vi "Startup Panel.vi"() -> (0 "Bool Out":bool, 1 "ROV Selector Out":u16, 2 "Port Number Recv Out 1":u16, 3 "IP Address Out":string, 4 "Restart Out":bool, 6 "Port Number  Send Out":u16, 8 "Port Number Joyst. Out":u16)   [LabVIEW 2014]
uses:
  <vilib>/Platform/TimedLoop/XDataNode/timing_clust.ctl
  <vilib>/Platform/TimedLoop/XDataNode/nitl_modes.ctl
  <vilib>/Platform/TimedLoop/XDataNode/wakeup.ctl
  <vilib>/Platform/TimedLoop/XDataNode/XDataNode.xnode
  <vilib>/Platform/TimedLoop/XDataNode/XDNodeRunTimeDep.lvlib
panel:
  in  "Port Number Joyst.":u16=8520
  in  "Port Number  Send":u16=8510
  in  "Restart":bool
  in  "Cancel Button":bool
  in  "OK Button":bool
  in  "ROV Selector":u16(ring) items=["Minerva", "Neptune"]
  in  "Port Number Recv":u16=8500
  in  "IP Address":string="localhost"
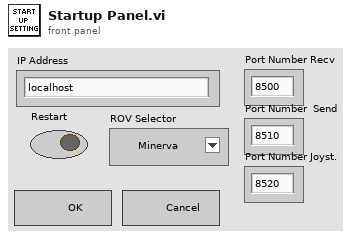
[diagram p1: front panel]
types:
  T1 = typedef "XDNodeRunTimeDep.lvlib/timing_clust.ctl" = cluster{"Expected End [f-1]":u64, "Actual End [f-1]":u64, "Finished Late? [f-1]":bool, "Expected End [i-1]":u64, "Actual End [i-1]":u64, "Finished Late? [i-1]":bool, "Expected Start [i]":u64, "Actual Start [i]":u64, "Expected Start [f]":u64, "Actual Start [f]":u64, "Source Name":string, "Structure Name":string, "Period":i64, "Deadline":i64, "Offset":i64, "Start":i64, "Priority":i32, "Timeout":i32, "Mode":T2, "Wakeup Reason":T3, "Error":errorcluster, "Source Type":string, "Secondary Source Type":string, "Global End Time":u64, "Global Start Time":u64, "Frame Duration":u64, "Iteration Duration":u64, "Assigned CPU":i32, "I/O Scan Engine Mode":u32}
  T2 = typedef "XDNodeRunTimeDep.lvlib/nitl_modes.ctl" = enum32{"No Change", "Process missed periods, maintain original phase", "Discard missed periods, maintain original phase", "Process missed periods, ignore original phase", "Discard missed periods, ignore original phase"}
  T3 = typedef "XDNodeRunTimeDep.lvlib/wakeup.ctl" = enum32{"Normal", "Aborted", "Asynchronous wakeup", "Timing source error", "Timed loop error", "Timeout"}
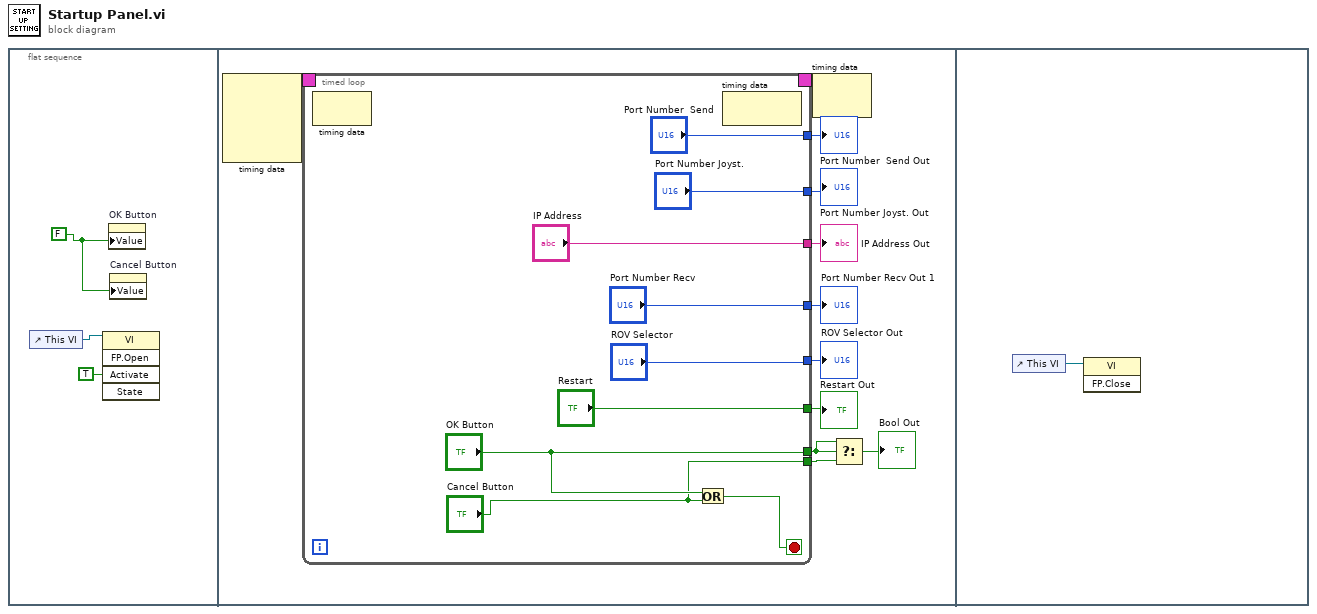
[diagram p0: block diagram]
diagram:
  n1 = flat-sequence {
    frame #0 {
      w1 = FALSE
      n2 = control-ref of="This VI"() -> (w3:refnum<vi>)
      n3 = invoke class="VI" method="FP.Open"(reference=w3, "Activate"=TRUE ("Activate?")) -> ()  [unwired: 3 in, 5 out]
      n4 = property on="OK Button" class="Bool (strict)"("Value"=w1) -> ()  [unwired: 2 in, 2 out]
      n5 = property on="Cancel Button" class="Bool (strict)"("Value"=w1) -> ()  [unwired: 2 in, 2 out]
    }
    frame #1 {
      n6 = node-c288() -> (w5:T1)  [unwired: 4 in]
      n7 = timed-loop {
        tunnel: ["IP Address"] -> w14
        tunnel: ["Port Number Recv"] -> w13
        tunnel: ["ROV Selector"] -> w12
        tunnel: ["OK Button"] -> w11
        tunnel: ["Cancel Button"] -> w10
        tunnel: ["Restart"] -> w8
        tunnel: ["Port Number  Send"] -> w6
        tunnel: ["Port Number Joyst."] -> w7
        timing: w5 -> [_]
        timing-out: [_] -> w4
        stop <- w23 stop-if-true
        n8 = node-c288() -> ()  [unwired: 1 in, 1 out]
        n9 = Or(x="OK Button", y="Cancel Button") -> (x .or. y?=w23:bool)
        n10 = node-c288() -> ()  [unwired: 1 in, 1 out]
      }
      "IP Address Out" <- w14
      "Port Number Recv Out 1" <- w13
      "ROV Selector Out" <- w12
      "Restart Out" <- w8
      "Port Number Joyst. Out" <- w7
      "Port Number  Send Out" <- w6
      n11 = node-c288(w4) -> ()  [unwired: 1 out]
      n12 = Select(t=w11, s=w11, f=w10) -> (s? t:f=→"Bool Out":bool)
    }
    frame #2 {
      n13 = control-ref of="This VI"() -> (w28:refnum<vi>)
      n14 = invoke class="VI" method="FP.Close"(reference=w28) -> ()  [unwired: 2 in, 3 out]
    }
  }
